vi "Get Caps Lock Key State.vi"(8 "Error In":errorcluster, 11 "path in":path) -> (0 "error out":errorcluster, 2 "Caps Lock Key State (Text)":string, 3 "Caps Lock Key State (Numeric)":i16 format="%02d")   [LabVIEW 2018]
doc: "Get Caps Lock Key State.vi\n\n<B>Description:</B>\nThe Get Caps Lock Key State VI returns the current state of the Caps Lock key.\n\nThe VI calls the Windows API (User32.dll) and uses the GetKeyState function to get the key state.\n \n<B>Inputs:</B>\nVK_CAPITAL - Virtual Key Code. VK_CAPITAL - 0x14 (CAPS LOCK key). For reference, a list of Virtual key codes can be found here: http://msdn.microsoft.com/en-us/library/windows/desktop/dd375731(v=vs.85).aspx \n\nerror in - Standard error cluster.\n\n<B>Outputs:</B>\nCaps Lock Key State (Numeric) - Current state of the Caps Lock key (Numeric).\n\n0 if the key is neither down nor toggled,\n\n-127 if the key is down and toggled,\n\n1 if the key is up and toggled, and\n\n-128 if the key is down but not toggled.\n\nA toggle key's indicator light (if any) on the keyboard will be on when the key is toggled, and off when the key is untoggled.\n\nCaps Lock Key State (Text) - Current state of the Caps Lock key (Text). A text description of the current Caps Lock key state.\n\nerror out - Standard error cluster.\n\n<B>Developed By:</B>\nMark Ridgley\nmark.ridgley_labview.developer@comcast.net"
panel:
  in  "VK_CAPITAL":i16=20
  # "For reference, a list of Virtual key codes can be found here: http://msdn.microsoft.com/en-us/library/windows/desktop/dd375731(v=vs.85).aspx"
  # "0 if the key is neither down nor toggled,\n\n-127 if the key is down and toggled,\n\n1 if the key is up and toggled, and\n\n-128 if the key is down but not toggled.\n\nA toggle key's indicator light (if any) on the keyboard will be on when the key is toggled, and off when the key is untoggled."
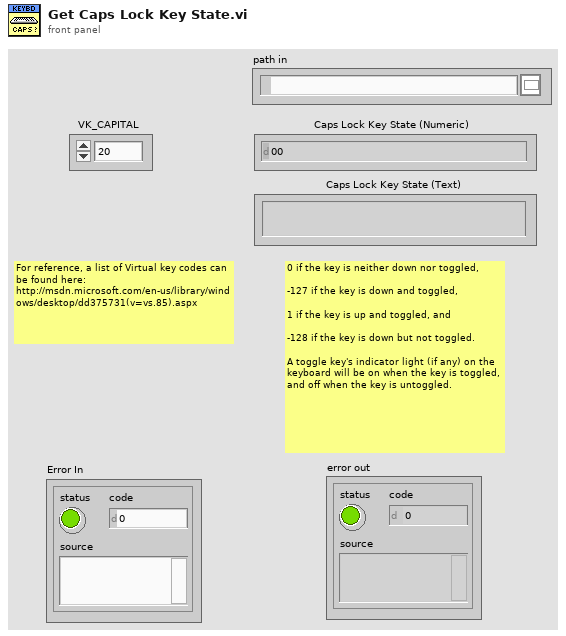
[diagram p1: front panel]
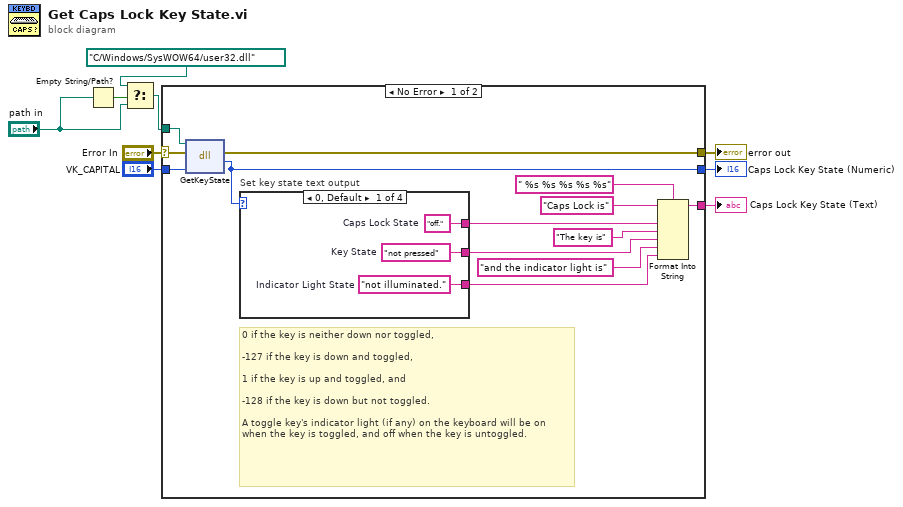
[diagram p0: block diagram]
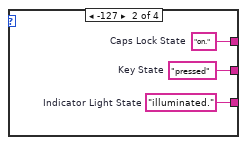
[diagram p2: hidden frame]
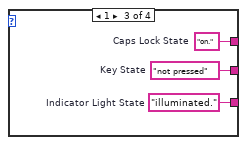
[diagram p3: hidden frame]
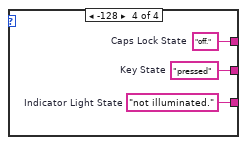
[diagram p4: hidden frame]
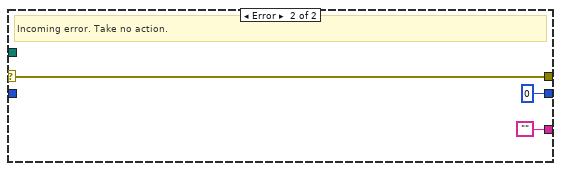
[diagram p5: hidden frame]
diagram:
  n1 = Empty String/Path?(string/path="path in") -> (empty?=w4:bool)
  n2 = Select(t=path "C:/Windows/SysWOW64/user32.dll" ("path in 2"), s=w4, f="path in") -> (s? t:f=w1:path)
  n3 = case shown="No Error" "Error In" {
    selector: "Error In" -> [w19 w37]
    tunnel: [w22 w37] -> w9
    tunnel: "VK_CAPITAL" -> [w21 _]
    tunnel: [w20 i16 0 ("return type")] -> w7
    tunnel: [w17 ""] -> w5
    tunnel: w1 -> [w10 _]
    frame No Error {
      # "0 if the key is neither down nor toggled,\n\n-127 if the key is down and toggled,\n\n1 if the key is up and toggled, and\n\n-128 if the key is down but not toggled.\n\nA toggle key's indicator light (if any) on the keyboard will be on when the key is toggled, and off when the key is untoggled."
      n4 = dll-call lib="C:/Windows/SysWOW64/user32.dll" fn="GetKeyState"(path in=w10, error in=w19, "nvirtkey"=w21) -> (error out=w22:errorcluster, "return type"=w20:i16)  [unwired: 2 in, 1 out]
      n5 = case "Set key state text output" shown="0, Default" w20 {
        tunnel: [w25 w28 w31 w34] -> w16
        tunnel: [w24 w27 w30 w33] -> w14
        tunnel: [w23 w26 w29 w32] -> w13
        frame 0, Default {
          w23 = "not illuminated."  # Indicator Light State
          w24 = "not pressed"  # Key State
          w25 = "off."  # Caps Lock State
        }
        frame -127 {
          w26 = "illuminated."  # Indicator Light State
          w27 = "pressed"  # Key State
          w28 = "on."  # Caps Lock State
        }
        frame 1 {
          w29 = "illuminated."  # Indicator Light State
          w30 = "not pressed"  # Key State
          w31 = "on."  # Caps Lock State
        }
        frame -128 {
          w32 = "not illuminated."  # Indicator Light State
          w33 = "pressed"  # Key State
          w34 = "off."  # Caps Lock State
        }
      }
      n6 = Format Into String(format string=" %s %s %s %s %s", initial string="Caps Lock is", w16, "The key is", w14, "and the indicator light is", w13) -> (resulting string=w17:string)  [unwired: 1 in, 1 out]
    }
    frame Error {
      # "Incoming error. Take no action."
    }
  }
  "error out" <- w9
  "Caps Lock Key State (Numeric)" <- w7
  "Caps Lock Key State (Text)" <- w5
